vi "AIP module.vi"(6 "Imaging Parameter.Line Averages":u8, 7 "Manual Controls.PSOCT Channel":u32, 8 "Y":i32=1100, 9 "X":i32=1100, 10 "Z":i32=100, 11 "3D volume":sgl[](array[numeric])) -> (2 "AIP":sgl[][](array[numeric]), 3 "Bline":dbl[][](array[numeric]))   [LabVIEW 2018]
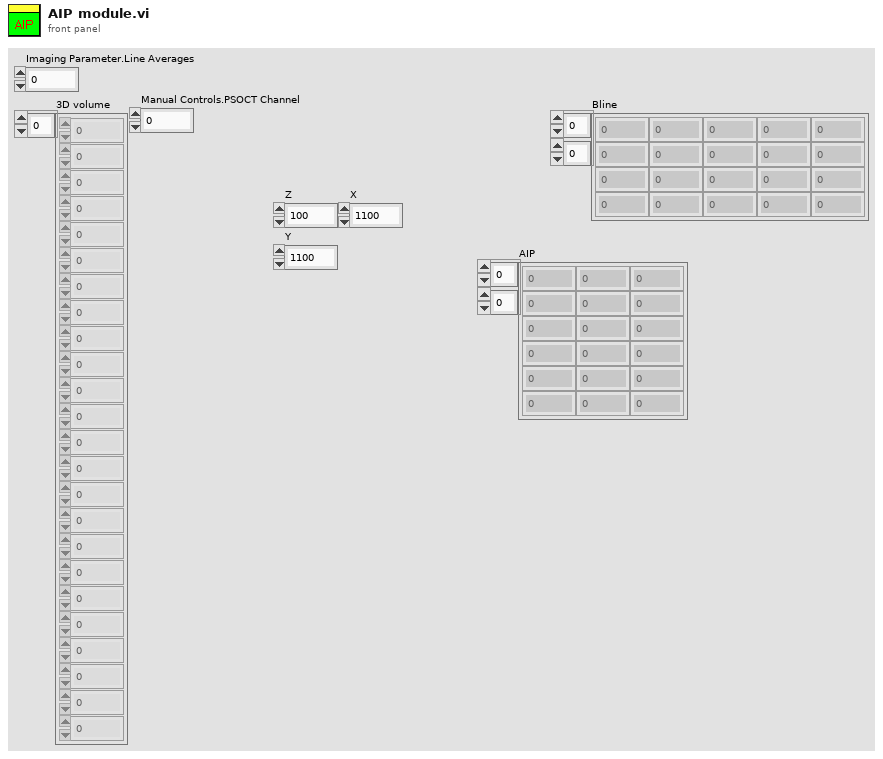
[diagram p1: front panel]
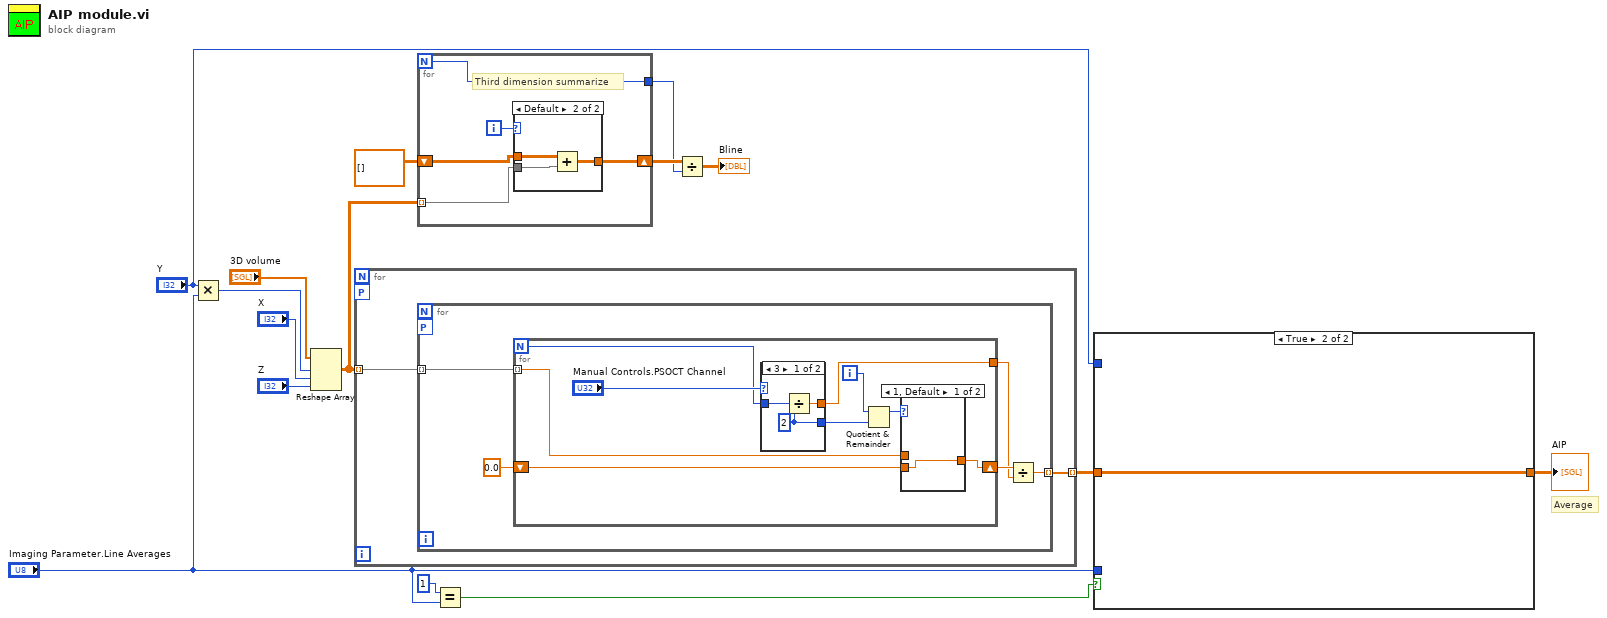
[diagram p0: block diagram]
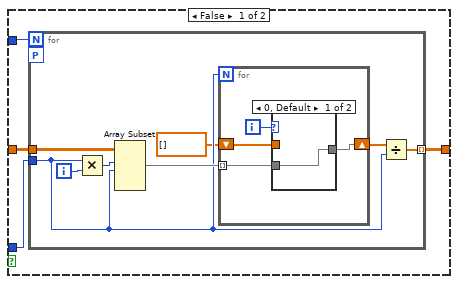
[diagram p2: hidden frame]
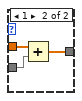
[diagram p3: hidden frame]
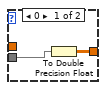
[diagram p4: hidden frame]
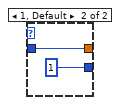
[diagram p5: hidden frame]
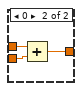
[diagram p6: hidden frame]
diagram:
  # "Average"
  n1 = Multiply(x="Y", y="Imaging Parameter.Line Averages") -> (x*y=w8:i32)
  n2 = Reshape Array("3D volume", w8, "X", "Z") -> (w1:sgl[][][])
  n3 = for {
    tunnel: w1 -> [w17] mode=indexing
    tunnel: [w16] -> w4 mode=indexing
    workers-P: _ -> [_]
    n4 = for {
      tunnel: w17 -> [w22] mode=indexing
      tunnel: [w19] -> w16 mode=indexing
      workers-P: _ -> [_]
      n5 = for {
        N -> [w24]
        tunnel: w22 -> [w31] mode=indexing
        shift-right: [w29] -> w21
        shift-left: sgl 0.0 -> [w30]
        tunnel: [w23] -> w20
        i -> [w28]
        n6 = case shown="3" "Manual Controls.PSOCT Channel" {
          tunnel: [w34 1 ("y")] -> w27
          tunnel: w24 -> [w33 w35]
          tunnel: [w32 w35] -> w23
          frame 3 {
            w34 = 2 ("y")
            n7 = Divide(x=w33, y=w34) -> (x/y=w32:dbl)
          }
          frame 1, Default {
          }
        }
        n8 = Quotient & Remainder(x=w28, y=w27) -> (x-y*floor(x/y)=w26:i32)  [unwired: 1 out]
        n9 = case shown="1, Default" w26 {
          tunnel: w31 -> [_ w40]
          tunnel: w30 -> [w37 w39]
          tunnel: [w37 w38] -> w29
          frame 1, Default {
          }
          frame 0 {
            n10 = Add(x=w40, y=w39) -> (x+y=w38:sgl)
          }
        }
      }
      n11 = Divide(x=w21, y=w20) -> (x/y=w19:dbl)
    }
  }
  n12 = for {
    N -> [w42]
    shift-right: [w45] -> w11
    shift-left: sgl[][] [] -> [w44]
    tunnel: [w42] -> w10
    tunnel: w1 -> [w41] mode=indexing
    i -> [w43]
    # "Third dimension summarize"
    n13 = case shown="Default" w43 {
      tunnel: [w47 w50] -> w45
      tunnel: w44 -> [_ w49]
      tunnel: w41 -> [w46 w48]
      frame 0 {
        n14 = To Double Precision Float(number=w46) -> (double precision float=w47:dbl[][])
      }
      frame Default {
        n15 = Add(x=w49, y=w48) -> (x+y=w50:dbl[][])
      }
    }
  }
  n16 = Equal?(x=u8 1, y="Imaging Parameter.Line Averages") -> (x = y?=w7:bool)
  n17 = Divide(x=w11, y=w10) -> (x/y=→"Bline":dbl[][])
  n18 = case shown="True" w7 {
    tunnel: [w51 w71] -> w5
    tunnel: w4 -> [w54 w71]
    tunnel: "Y" -> [w53 _]
    tunnel: "Imaging Parameter.Line Averages" -> [w52 _]
    frame False {
      n19 = for {
        N: w53 -> [_]
        tunnel: w54 -> [w61]
        tunnel: w52 -> [w57]
        tunnel: [w56] -> w51 mode=indexing
        workers-P: _ -> [_]
        i -> [w62]
        n20 = Multiply(x=w57, y=w62) -> (x*y=w60:i32)
        n21 = Array Subset(array=w61, index (row)=w60, length (row)=w57) -> (w59:dbl[][])  [unwired: 2 in]
        n22 = for {
          N: w57 -> [_]
          tunnel: w59 -> [w65] mode=indexing
          shift-right: [w64] -> w58
          shift-left: sgl[] [] -> [w63]
          i -> [w66]
          n23 = case shown="0, Default" w66 {
            tunnel: w65 -> [w67 w70]
            tunnel: [w67 w69] -> w64
            tunnel: w63 -> [_ w68]
            frame 0, Default {
            }
            frame 1 {
              n24 = Add(x=w68, y=w70) -> (x+y=w69:dbl[])
            }
          }
        }
        n25 = Divide(x=w58, y=w57) -> (x/y=w56:dbl[])
      }
    }
    frame True {
    }
  }
  "AIP" <- w5
